vi "Query Trace Data.vi"(8 "error in (no error)":errorcluster, 11 "SA-FSW in":refnum<class "SA-FSW.lvclass">) -> (0 "error out":errorcluster, 1 "Level":dbl[](array[numeric]), 2 "Frequency/Time":dbl[](array[numeric]), 3 "SA-FSW out":refnum<class "SA-FSW.lvclass">)   [LabVIEW 2020, in "SA-FSW.lvclass"]
uses:
  SA-FSW.lvclass
  C:/Sandbox/RF Bench/Source Code/WiSpry Test Framework/Instruments/Instrument.lvclass
  C:/Sandbox/RF Bench/Source Code/WiSpry Test Framework/Instruments/Spectrum Analyzer/Spectrum Analyzer.lvclass
  Spectrum Analyzer.lvclass/Spectrum Analyzer.ctl
  Instrument.lvclass/Instrument.ctl
  Instrument.lvclass
  Spectrum Analyzer.lvclass
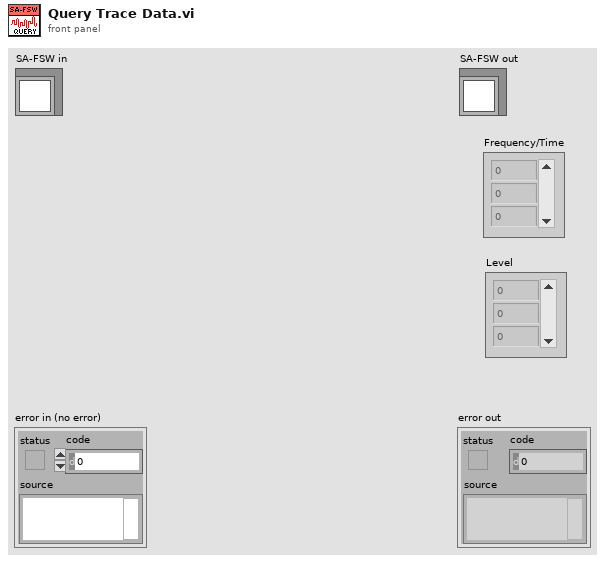
[diagram p1: front panel]
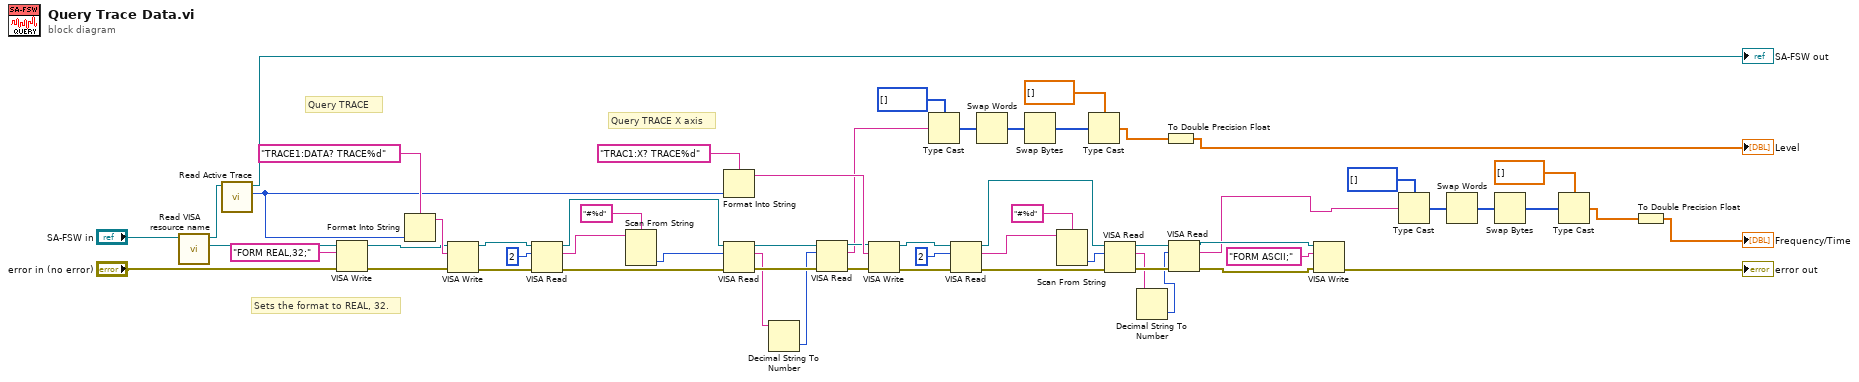
[diagram p0: block diagram]
diagram:
  # "Sets the format to REAL, 32."
  # "Query TRACE X axis"
  # "Query TRACE"
  n1 = call "Read VISA resource name.vi"("Instrument in"="SA-FSW in") -> ("VISA resource name"=w32:refnum<visa-resource-name>, "Instrument out"=w58:refnum<class "SA-FSW.lvclass">)  [unwired: 9 in]
  n2 = call "Read Active Trace.vi"("Spectrum Analyzer in"=w58) -> ("Active Trace"=w45:u16, "Spectrum Analyzer out"=→"SA-FSW out":refnum<class "SA-FSW.lvclass">)  [unwired: 9 in]
  n3 = VISA Write(VISA resource name=w32, write buffer="FORM REAL,32;", error in (no error)="error in (no error)") -> (VISA resource name out=w34:refnum<visa-resource-name>, error out=w35:errorcluster)  [unwired: 1 out]
  n4 = Format Into String(format string="TRACE1:DATA? TRACE%d", w45) -> (resulting string=w56:string)  [unwired: 2 in, 1 out]
  n5 = VISA Write(VISA resource name=w34, write buffer=w56, error in (no error)=w35) -> (VISA resource name out=w54:refnum<visa-resource-name>, error out=w55:errorcluster)  [unwired: 1 out]
  n6 = VISA Read(VISA resource name=w54, byte count=u32 2, error in (no error)=w55) -> (VISA resource name out=w49:refnum<visa-resource-name>, read buffer=w53:string, error out=w51:errorcluster)  [unwired: 1 out]
  n7 = Scan From String(format string="#%d", input string=w53) -> (output 1=w30:i32)  [unwired: 3 in, 3 out]
  n8 = Format Into String(format string="TRAC1:X? TRACE%d", w45) -> (resulting string=w47:string)  [unwired: 2 in, 1 out]
  n9 = VISA Read(VISA resource name=w49, byte count=w30, error in (no error)=w51) -> (VISA resource name out=w26:refnum<visa-resource-name>, read buffer=w25:string, error out=w27:errorcluster)  [unwired: 1 out]
  n10 = Decimal String To Number(string=w25) -> (number=w24:i32)  [unwired: 2 in, 1 out]
  n11 = VISA Read(VISA resource name=w26, byte count=w24, error in (no error)=w27) -> (VISA resource name out=w28:refnum<visa-resource-name>, read buffer=w16:string, error out=w29:errorcluster)  [unwired: 1 out]
  n12 = VISA Write(VISA resource name=w28, write buffer=w47, error in (no error)=w29) -> (VISA resource name out=w42:refnum<visa-resource-name>, error out=w43:errorcluster)  [unwired: 1 out]
  n13 = Type Cast(type=i32[] [], x=w16) -> (*(type *) &x=w14:i32[])
  n14 = VISA Read(VISA resource name=w42, byte count=u32 2, error in (no error)=w43) -> (VISA resource name out=w38:refnum<visa-resource-name>, read buffer=w39:string, error out=w40:errorcluster)  [unwired: 1 out]
  n15 = Swap Words(1:w14) -> (0:w13:i32[])
  n16 = Swap Bytes(anything=w13) -> (byte swapped=w12:i32[])
  n17 = Scan From String(format string="#%d", input string=w39) -> (output 1=w23:i32)  [unwired: 3 in, 3 out]
  n18 = Type Cast(type=sgl[] [], x=w12) -> (*(type *) &x=w10:sgl[])
  n19 = VISA Read(VISA resource name=w38, byte count=w23, error in (no error)=w40) -> (VISA resource name out=w21:refnum<visa-resource-name>, read buffer=w18:string, error out=w22:errorcluster)  [unwired: 1 out]
  n20 = Decimal String To Number(string=w18) -> (number=w17:i32)  [unwired: 2 in, 1 out]
  n21 = To Double Precision Float(number=w10) -> (double precision float=→"Level":dbl[])
  n22 = VISA Read(VISA resource name=w21, byte count=w17, error in (no error)=w22) -> (VISA resource name out=w20:refnum<visa-resource-name>, read buffer=w2:string, error out=w19:errorcluster)  [unwired: 1 out]
  n23 = VISA Write(VISA resource name=w20, write buffer="FORM ASCII;", error in (no error)=w19) -> (error out=→"error out":errorcluster)  [unwired: 2 out]
  n24 = Type Cast(type=i32[] [], x=w2) -> (*(type *) &x=w4:i32[])
  n25 = Swap Words(1:w4) -> (0:w5:i32[])
  n26 = Swap Bytes(anything=w5) -> (byte swapped=w6:i32[])
  n27 = Type Cast(type=sgl[] [], x=w6) -> (*(type *) &x=w8:sgl[])
  n28 = To Double Precision Float(number=w8) -> (double precision float=→"Frequency/Time":dbl[])
